vi "Create Currency Map.vi"() -> (0 "error out":errorcluster, 2 "Value":dbl[](array[numeric]), 3 "Denomination":string[](array[string]))   [LabVIEW 2020, in "Config File Management.lvlib"]
doc: "Creates a map with the currency values and strings for buttons"
uses:
  Config File Management.lvlib
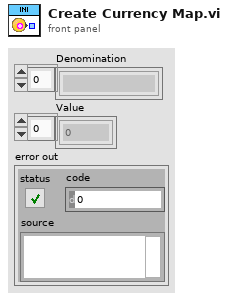
[diagram p1: front panel]
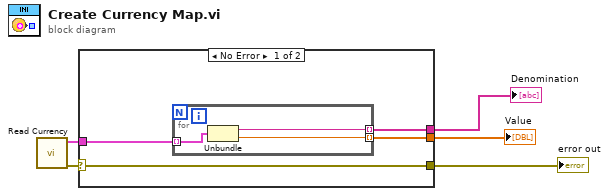
[diagram p0: block diagram]
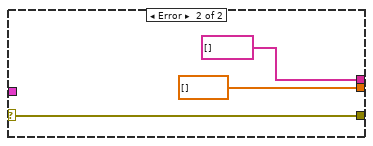
[diagram p2: hidden frame]
diagram:
  n1 = call "Read Currency.vi"() -> ("error out"=w4:errorcluster, "Array"=w5:cluster{"Denomination":string, "Value":dbl}[])  [unwired: 10 in]
  n2 = case shown="No Error" w4 {
    selector: w4 -> [w8 w14]
    tunnel: w5 -> [w9 _]
    tunnel: [w8 w14] -> w1
    tunnel: [w7 string[] []] -> w3
    tunnel: [w6 dbl[] []] -> w2
    frame No Error {
      n3 = for {
        tunnel: w9 -> [w12] mode=indexing
        tunnel: [w11] -> w7 mode=indexing
        tunnel: [w10] -> w6 mode=indexing
        n4 = Unbundle(w12) -> ("Denomination"=w11:string, "Value"=w10:dbl)
      }
    }
    frame Error {
    }
  }
  "Denomination" <- w3
  "Value" <- w2
  "error out" <- w1
